vi "Teleope Balance 3.vi"(9 "Start Time":dbl, 10 "Button":bool) -> ()   [LabVIEW 2020]
uses:
  Robot Global Data.vi
  <vilib>/Rock Robotics/WPI/Utilities/WPI_GetSetVariantRefNum.vi
  <vilib>/Rock Robotics/WPI/RobotDrive/WPI_RobotDriveArcadeDrive_Standard(NoSaturation).vi
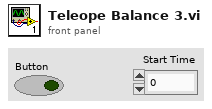
[diagram p1: front panel]
types:
  T1 = typedef "WPI_RobotDriveDevRef.ctl" = cluster{"DevStatus":errorcluster, "Motors[]":T2[], "Square Inputs":bool, "Max Output":dbl}
  T2 = typedef "WPI_MotorControlDeviceRef.ctl" = cluster{"DeviceStatus":errorcluster, "Type":T3, "PWM":cluster{"PWM Channel":T4, "DeadBand":T5}, "CAN":cluster{"Device Number":u8, "SetOutput VI Ref":variant, "GetOutput VI Ref":variant, "Enable VI Ref":variant, "Disable VI Ref":variant, "Data":variant}, "Invert":bool, "DIO PWM":cluster{"PWM \"Enable\" Channel":T4, "DIOChannel":T6, "PWM Rate":dbl}}
  T3 = typedef "WPI_MotorControlType.ctl" = enum16{"PWM", "CAN", "DIO PWM"}
  T4 = typedef "FPGA_DIOPWMChannel.ctl" = enum8{"PWM 0", "PWM 1", "PWM 2", "PWM 3", "PWM 4", "PWM 5", "PWM 6", "PWM 7", "PWM 8", "PWM 9", "PWM MXP 0", "PWM MXP 1", "PWM MXP 2", "PWM MXP 3", "PWM MXP 4", "PWM MXP 5", "PWM MXP 6", "PWM MXP 7", "PWM MXP 8", "PWM MXP 9", "Invalid"}
  T5 = typedef "WPI_PWMDeadband.ctl" = cluster{"Name":string, "maxPositivePwm":i32, "minPositivePwm":i32, "centerPwm":i32, "maxNegativePwm":i32, "minNegativePwm":i32, "angularRange":u16}
  T6 = typedef "FPGA_DIOChannel.ctl" = enum8{"DIO 0", "DIO 1", "DIO 2", "DIO 3", "DIO 4", "DIO 5", "DIO 6", "DIO 7", "DIO 8", "DIO 9", "DIO MXP 0", "DIO MXP 1", "DIO MXP 2", "DIO MXP 3", "DIO MXP 4", "DIO MXP 5", "DIO MXP 6", "DIO MXP 7", "DIO MXP 8", "DIO MXP 9", "DIO MXP 10", "DIO MXP 11", "DIO MXP 12", "DIO MXP 13", "DIO MXP 14", "DIO MXP 15", "SPI Port CS1", "SPI Port CS2", "SPI Port CS3", "SPI Port MISO", "SPI Port MOSI", "Invalid"}
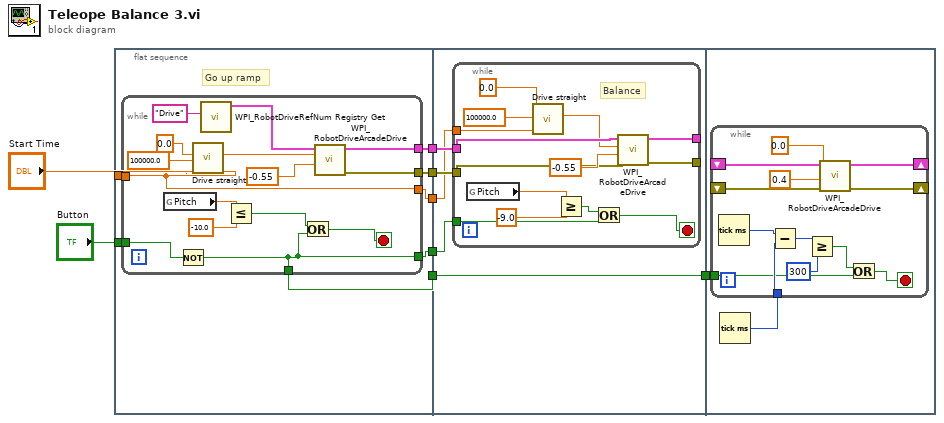
[diagram p0: block diagram]
diagram:
  n1 = flat-sequence {
    tunnel: [w15] -> w8
    tunnel: [w14] -> w7
    tunnel: "Start Time" -> [w13]
    tunnel: [w12] -> w6
    tunnel: "Button" -> [w11]
    tunnel: [w10] -> w3
    tunnel: [w9] -> w1
    tunnel: w8 -> [w35]
    tunnel: w7 -> [w34]
    tunnel: w6 -> [w33]
    tunnel: w3 -> [w32]
    tunnel: [w31] -> w2
    tunnel: w1 -> [w31]
    tunnel: w2 -> [w50]
    frame #0 {
      # "Go up ramp"
      n2 = while {
        tunnel: [w25] -> w15
        tunnel: [w24] -> w14
        tunnel: w13 -> [w20]
        tunnel: [w20] -> w12
        tunnel: w11 -> [w19]
        tunnel: [w16] -> w10
        tunnel: [w16] -> w9
        stop <- w17 stop-if-true
        n3 = global read "Robot Global Data.vi" "Pitch"() -> (w27:dbl)
        n4 = Not(x=w19) -> (.not. x?=w16:bool)
        n5 = call "Drive straight.vi"("Start Time"=w20, "Length(seconds)"=100000.0, "Desired angle"=0.0) -> ("X Power"=w23:dbl)  [unwired: 7 in, 1 out]
        n6 = call <vilib>:"WPI_RobotDriveRefNum Registry Get.vi"("refnum name"="Drive") -> ("RobotDriveDevRef"=w29:T1)  [unwired: 9 in, 1 out]
        n7 = Less Or Equal?(x=w27, y=-10.0) -> (x <= y?=w18:bool)
        n8 = Or(x=w18, y=w16) -> (x .or. y?=w17:bool)
        n9 = call-poly <vilib>:"WPI_RobotDriveArcadeDrive.vi"("Y axis value"=-0.55, "X axis value"=w23, "RobotDriveDevRef"=w29) -> ("error out"=w24:errorcluster, "RobotDriveDevRef"=w25:T1)  [unwired: 6 in, 1 out]
      }
    }
    frame #1 {
      n10 = while {
        tunnel: [w47] -> _
        tunnel: w35 -> [w46]
        tunnel: w34 -> [w45]
        tunnel: [w43] -> _
        tunnel: w33 -> [w40]
        tunnel: w32 -> [w36]
        stop <- w37 stop-if-true
        # "Balance"
        n11 = global read "Robot Global Data.vi" "Pitch"() -> (w44:dbl)
        n12 = call "Drive straight.vi"("Start Time"=w40, "Length(seconds)"=100000.0, "Desired angle"=0.0) -> ("X Power"=w41:dbl)  [unwired: 7 in, 1 out]
        n13 = Greater Or Equal?(x=w44, y=-9.0) -> (x >= y?=w38:bool)
        n14 = Or(x=w38, y=w36) -> (x .or. y?=w37:bool)
        n15 = call-poly <vilib>:"WPI_RobotDriveArcadeDrive.vi"("error in (no error)"=w45, "Y axis value"=-0.55, "X axis value"=w41, "RobotDriveDevRef"=w46) -> ("error out"=w43:errorcluster, "RobotDriveDevRef"=w47:T1)  [unwired: 5 in, 1 out]
      }
    }
    frame #2 {
      n16 = Tick Count (ms)() -> (millisecond timer value=w51:u32)
      n17 = while {
        shift-right: [w62] -> _
        shift-left: _ -> [w64]
        shift-right: [w61] -> _
        shift-left: _ -> [w63]
        tunnel: w51 -> [w57]
        tunnel: w50 -> [w52]
        stop <- w53 stop-if-true
        n18 = Tick Count (ms)() -> (millisecond timer value=w58:u32)
        n19 = Subtract(x=w58, y=w57) -> (x-y=w56:u32)
        n20 = Greater Or Equal?(x=w56, y=u32 300) -> (x >= y?=w54:bool)
        n21 = call-poly <vilib>:"WPI_RobotDriveArcadeDrive.vi"("error in (no error)"=w63, "Y axis value"=0.4, "X axis value"=0.0, "RobotDriveDevRef"=w64) -> ("error out"=w61:errorcluster, "RobotDriveDevRef"=w62:T1)  [unwired: 5 in, 1 out]
        n22 = Or(x=w54, y=w52) -> (x .or. y?=w53:bool)
      }
    }
  }
